vi "SelectData.vi"(0 "SQL query":string="select * from t_sample_info;", 3 "error in":errorcluster) -> (6 "recordset data":variant[][](array[variant]), 9 "error out":errorcluster)   [LabVIEW 2014, in "DataBase.lvlib"]
uses:
  DataBase.lvlib
  <vilib>/addons/database/Connection.llb/DB Tools Open Connec (String).vi
  <vilib>/addons/database/Connection.llb/Conn Execute.vi
  <vilib>/addons/database/Recordset.llb/Rec Fetch Recordset Data (R).vi
  <vilib>/addons/database/Recordset.llb/Rec Destroy - Connection.vi
  <vilib>/addons/database/NI_Database_API.lvlib
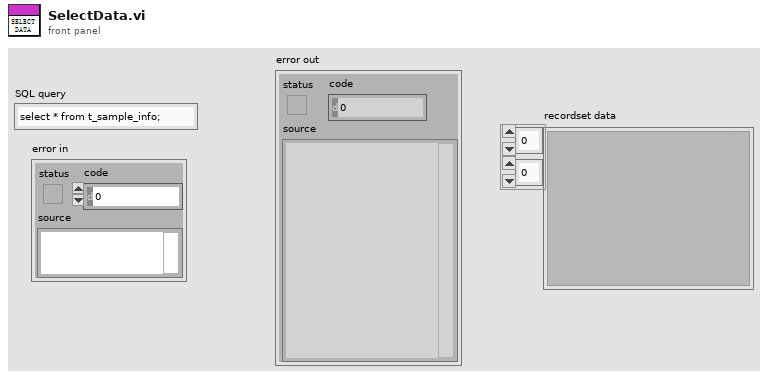
[diagram p1: front panel]
types:
  T1 = typedef "NI_Database_API.lvlib/Conn ObjectReference.ctl" = refnum<k1>
  T2 = typedef "NI_Database_API.lvlib/Rec ObjectReference.ctl" = refnum<k1>
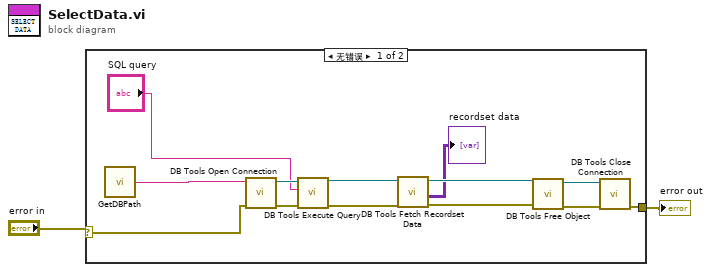
[diagram p0: block diagram]
diagram:
  n1 = case shown="无错误" "error in" {
    selector: "error in" -> [w11 w16]
    tunnel: [w10 w16] -> w1
    frame No Error {
      n2 = call "GetDBPath.vi"() -> ("Connection"=w9:string)  [unwired: 1 in]
      n3 = call-poly <vilib>:"DB Tools Open Connection.vi"("error in (no error)"=w11, "connection information"=w9) -> ("error out"=w14:errorcluster, "connection reference"=w15:T1)  [unwired: 6 in]
      n4 = call-poly <vilib>:"DB Tools Execute Query.vi"("error in (no error)"=w14, "SQL query"="SQL query", "connection reference"=w15) -> ("error out"=w7:errorcluster, "recordset reference"=w6:T2)  [unwired: 5 in]
      n5 = call-poly <vilib>:"DB Tools Fetch Recordset Data.vi"("error in (no error)"=w7, "recordset reference"=w6) -> ("error out"=w4:errorcluster, "recordset data"=→"recordset data":variant[][], "recordset reference out"=w5:T2)  [unwired: 3 in]
      n6 = call-poly <vilib>:"DB Tools Free Object.vi"("error in (no error)"=w4, "recordset reference"=w5) -> ("error out"=w13:errorcluster, "connection reference"=w12:T1)  [unwired: 8 in]
      n7 = call <vilib>:"DB Tools Close Connection.vi"("error in (no error)"=w13, "connection reference"=w12) -> ("error out"=w10:errorcluster)  [unwired: 5 in]
    }
    frame Error {
    }
  }
  "error out" <- w1
